vi "getpagesize.vi"(8 "error in (no error)":errorcluster) -> (0 "error out":errorcluster, 3 "page size":u32)   [LabVIEW 2013, in "Linux RT IPC.C.lvlib"]
doc: "Wrapper VI for Linux function getpagesize()."
uses:
  Linux RT IPC.C.lvlib
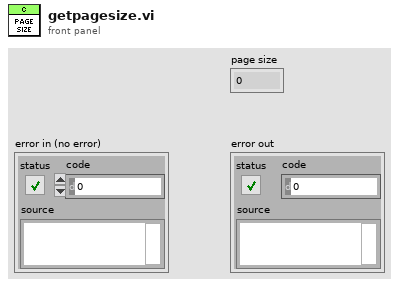
[diagram p1: front panel]
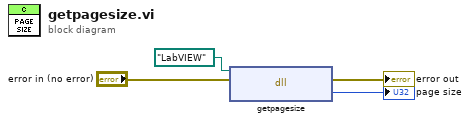
[diagram p0: block diagram]
diagram:
  n1 = dll-call lib="?" fn="getpagesize"(path in=path "LabVIEW", error in="error in (no error)") -> (error out=→"error out":errorcluster, "page size"=→"page size":u32)  [unwired: 1 in, 1 out]
